vi "Insert Test Step.vi"(8 "error in (no error)":errorcluster, 10 "Insert Test Step":T1, 11 "Test Executive Builder in":refnum<class "Test Executive Builder.lvclass">) -> (0 "error out":errorcluster, 3 "Test Executive Builder out":refnum<class "Test Executive Builder.lvclass">, 5 "Unique ID out":string)   [LabVIEW 2019, in "Test Executive Builder.lvclass"]
uses:
  <vilib>/gpm_packages/@cs/Test-executive-builder/Example/Application/Test Executive Builder/Test Executive Builder/Test Executive Builder.lvclass
  C:/Program Files/National Instruments/LabVIEW 2019/vi.lib/gpm_packages/@cs/Test-executive-builder/Source/Test Executive Builder Model/Test Executive Builder Model/Test Executive Builder Model.lvclass
  <vilib>/gpm_packages/@cs/Test-executive-builder/Source/Application Dependencies/Insert Test Step.ctl
  <vilib>/gpm_packages/@cs/Test-executive-builder/Example/Application/Test Executive Builder/Test Executive Builder/Test Executive Builder.lvclass/Test Executive Builder.ctl
  <vilib>/gpm_packages/@cs/Test-executive-builder/Source/Test Executive Builder Model/Test Executive Builder Model/Test Executive Builder Model.lvclass/Test Executive Builder Model.ctl
  cb65339b-8f39-4431-a9a5-95b4e30619be.vi
  <vilib>/Utility/error.llb/Error Cluster From Error Code.vi
  <vilib>/gpm_packages/@cs/Test-executive-builder/Source/Test Executive Builder Model/Test Executive Builder Model/Test Executive Builder Model.lvclass
  <vilib>/gpm_packages/@cs/test-executive/Source/Test Executive/ITestExecutive/ITest Executive.lvclass
  C:/Program Files/National Instruments/LabVIEW 2019/vi.lib/gpm_packages/@cs/mva-core/Source/IModel/IModel/IModel.lvclass
  C:/Program Files/National Instruments/LabVIEW 2019/vi.lib/gpm_packages/@cs/mva-core/Source/IObserver/IObserver/IObserver.lvclass
  C:/Program Files/National Instruments/LabVIEW 2019/vi.lib/ActorFramework/Actor/Actor.lvclass
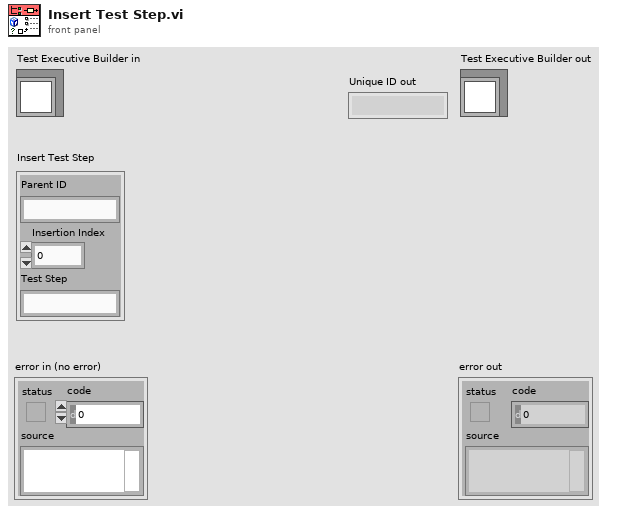
[diagram p1: front panel]
types:
  T1 = typedef "Insert Test Step.ctl" = cluster{"Parent ID":string, "Insertion Index":i32, "Test Step":string}
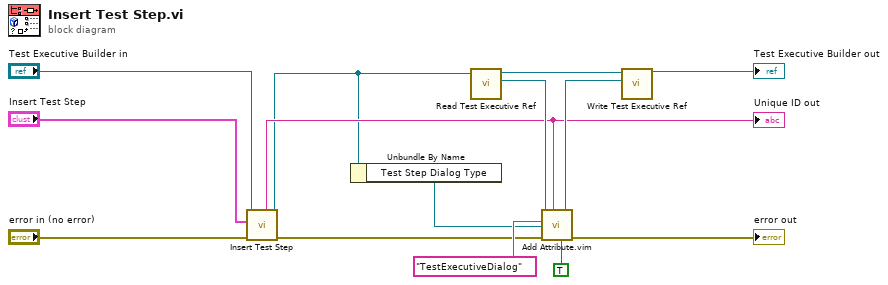
[diagram p0: block diagram]
diagram:
  n1 = call-parent "Insert Test Step.vi"("error in (no error)"="error in (no error)", "Insert Test Step"="Insert Test Step", "Test Executive Builder Model in"="Test Executive Builder in") -> ("error out"=w3:errorcluster, "Test Executive Builder Model out"=w1:refnum<class "Test Executive Builder.lvclass">, "Unique ID out"=w6:string)  [unwired: 6 in]
  "Unique ID out" <- w6
  n2 = Unbundle By Name(w1) -> ("Test Step Dialog Type"=w4:refnum<class "ITest Executive Builder Dialog.lvclass">)
  n3 = call <vilib>:"Read Test Executive Ref.vi"("Test Executive Builder Model in"=w1) -> ("Test Executive Ref"=w12:refnum<data-value>, "Test Executive Builder Model out"=w8:refnum<class "Test Executive Builder.lvclass">)  [unwired: 9 in]
  n4 = call "Add Attribute.vim"("Private?"=TRUE, "ID"=w6, "error in (no error)"=w3, "Attribute"=w4, "Attribute Name"="TestExecutiveDialog", "Test Executive Ref"=w12) -> ("error out"=→"error out":errorcluster, "Test Executive Ref out"=w11:refnum<data-value>)  [unwired: 2 in, 2 out]
  n5 = call <vilib>:"Write Test Executive Ref.vi"("Test Executive Ref"=w11, "Test Executive Builder Model in"=w8) -> ("Test Executive Builder Model out"=→"Test Executive Builder out":refnum<class "Test Executive Builder.lvclass">)  [unwired: 9 in]
